vi "InitaliseDAQ.vi"() -> (0 "Channels":T1)   [LabVIEW 2016]
uses:
  controls/PinOut.ctl
  <vilib>/DAQmx/create/channels.llb/DAQmx Create Channel (DO-Digital Output).vi
  <vilib>/DAQmx/create/channels.llb/DAQmx Create Channel (AO-Voltage-Basic).vi
panel:
  out "Analogue Out":refnum<k21>
  out "Digital Out":refnum<k21>
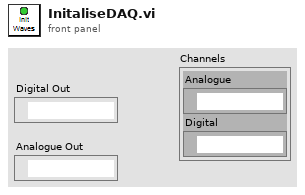
[diagram p1: front panel]
types:
  T1 = cluster{"Analogue":refnum<k21>, "Digital":refnum<k21>}
  T2 = typedef "PinOut.ctl" = string
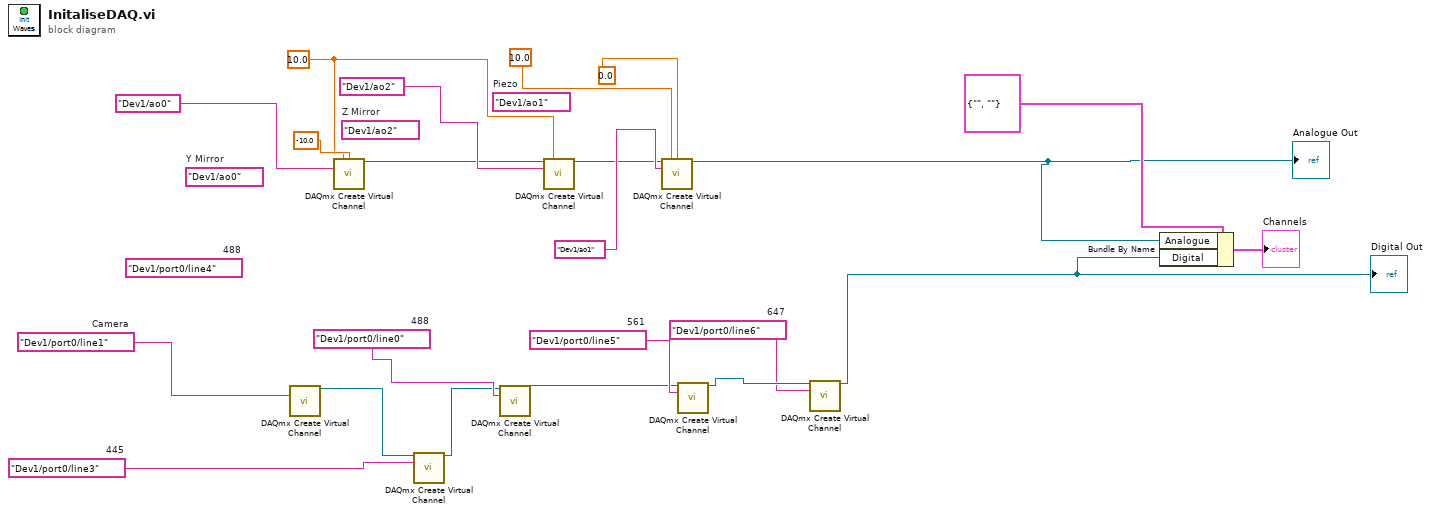
[diagram p0: block diagram]
diagram:
  (unwired) tag "Dev1/port0/line4"  # 488
  (unwired) tag "Dev1/ao1"  # Piezo
  (unwired) tag "Dev1/ao2"  # Z Mirror
  (unwired) tag "Dev1/ao0"  # Y Mirror
  w14 = 10.0 ("maximum value")
  w12 = tag "Dev1/port0/line6"  # 647
  w10 = tag "Dev1/port0/line5"  # 561
  w5 = tag "Dev1/port0/line3"  # 445
  w8 = tag "Dev1/port0/line0"  # 488
  w11 = tag "Dev1/port0/line1"  # Camera
  n1 = call-poly <vilib>:"DAQmx Create Virtual Channel.vi"("lines"=w11) -> ("task out"=w6:refnum<k21>)  [unwired: 13 in, 1 out]
  n2 = call-poly <vilib>:"DAQmx Create Virtual Channel.vi"("maximum value"=w14, "minimum value"=-10.0, "physical channels"=T2 "Dev1/ao0" ("Combo Box")) -> ("task out"=w18:refnum<k21>)  [unwired: 11 in, 1 out]
  n3 = call-poly <vilib>:"DAQmx Create Virtual Channel.vi"("task in"=w6, "lines"=w5) -> ("task out"=w7:refnum<k21>)  [unwired: 12 in, 1 out]
  n4 = call-poly <vilib>:"DAQmx Create Virtual Channel.vi"("task in"=w7, "lines"=w8) -> ("task out"=w9:refnum<k21>)  [unwired: 12 in, 1 out]
  n5 = call-poly <vilib>:"DAQmx Create Virtual Channel.vi"("task in"=w18, "maximum value"=w14, "physical channels"=T2 "Dev1/ao2" ("Combo Box")) -> ("task out"=w19:refnum<k21>)  [unwired: 11 in, 1 out]
  n6 = call-poly <vilib>:"DAQmx Create Virtual Channel.vi"("task in"=w19, "maximum value"=10.0 ("minimum value"), "minimum value"=0.0 ("maximum value"), "physical channels"=T2 "Dev1/ao1" ("Combo Box")) -> ("task out"=w3:refnum<k21>)  [unwired: 10 in, 1 out]
  "Analogue Out" <- w3
  n7 = call-poly <vilib>:"DAQmx Create Virtual Channel.vi"("task in"=w9, "lines"=w10) -> ("task out"=w13:refnum<k21>)  [unwired: 12 in, 1 out]
  n8 = call-poly <vilib>:"DAQmx Create Virtual Channel.vi"("task in"=w13, "lines"=w12) -> ("task out"=w2:refnum<k21>)  [unwired: 12 in, 1 out]
  "Digital Out" <- w2
  n9 = Bundle By Name(cluster=T1 {"Analogue"="", "Digital"=""} ("input cluster"), "Analogue"=w3, "Digital"=w2) -> (→"Channels":T1)
